vi "CRYTest and Insert CRY6181 Audio Channels.vi"(11 "Hardware in":T1={"Name"="", "Analog I/O"=0, "Digital I/O"=0, "Channels"=2, "Dig Dev ID"=1, "N ports"=3, "Interface"=0, "Dig I/O Ports"=[{"port #"=1, "width"=8, "direction"=0}, {"port #"=2, "width"=8, "direction"=0}, {"port #"=3, "width"=8, "direction"=0}], "Interf settings"=[], "N interfs"=3, "udev SNs"=[], "udev enable"=FALSE, "Channel Array"=[], "Cal sequence"="", "SelectedIn"=0, "SelectedOut"=0, "SelectedTab"=0, "State"=FALSE, "Help"="", "Advanced"=FALSE, "In Audio Driver"=0, "Out Audio Driver"=0} {"Channel Array"."Coupling" items=["Default"=-1, "RSE"=10083, "NRSE"=10078, "Differential"=10106, "Pseudodifferential"=12529]; "Channel Array"."term config" items=["Default"=-1, "RSE"=10083, "NRSE"=10078, "Differential"=10106, "Pseudodifferential"=12529]; "Channel Array"."Anti-aliasing Factor (%fs)" format="%.2f"}) -> (0 "Inserted channels":bool, 3 "Hardware out":T1={"Name"="", "Analog I/O"=0, "Digital I/O"=0, "Channels"=2, "Dig Dev ID"=1, "N ports"=3, "Interface"=0, "Dig I/O Ports"=[{"port #"=1, "width"=8, "direction"=0}, {"port #"=2, "width"=8, "direction"=0}, {"port #"=3, "width"=8, "direction"=0}], "Interf settings"=[], "N interfs"=3, "udev SNs"=[], "udev enable"=FALSE, "Channel Array"=[], "Cal sequence"="", "SelectedIn"=0, "SelectedOut"=0, "SelectedTab"=0, "State"=FALSE, "Help"="", "Advanced"=FALSE, "In Audio Driver"=0, "Out Audio Driver"=0} {"Channel Array"."Coupling" items=["Default"=-1, "RSE"=10083, "NRSE"=10078, "Differential"=10106, "Pseudodifferential"=12529]; "Channel Array"."term config" items=["Default"=-1, "RSE"=10083, "NRSE"=10078, "Differential"=10106, "Pseudodifferential"=12529]; "Channel Array"."Anti-aliasing Factor (%fs)" format="%.2f"})   [LabVIEW 2013]
uses:
  Typedef Control/CRYHardware.ctl
  Typedef Control/CRYHardware Channel Info.ctl
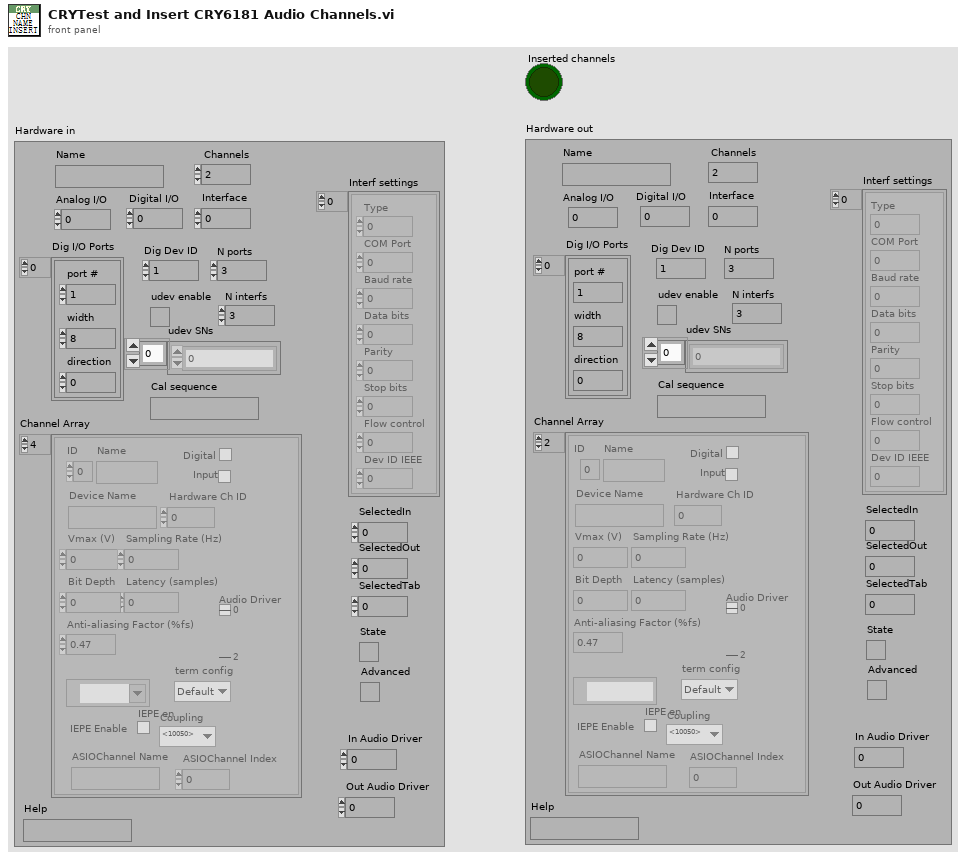
[diagram p1: front panel]
types:
  T1 = typedef "CRYHardware.ctl" = cluster{"Name":string, "Analog I/O":u16, "Digital I/O":u16, "Channels":u8, "Dig Dev ID":u8, "N ports":u8, "Interface":u32, "Dig I/O Ports":cluster{"port #":i16, "width":i16, "direction":i32}[], "Interf settings":cluster{"Type":u16, "COM Port":u8, "Baud rate":u32, "Data bits":u32, "Parity":u16, "Stop bits":u16, "Flow control":u16, "Dev ID IEEE":u8}[], "N interfs":i32, "udev SNs":i16[], "udev enable":bool, "Channel Array":T2[], "Cal sequence":string, "SelectedIn":u16, "SelectedOut":u16, "SelectedTab":u16, "State":bool, "Help":string, "Advanced":bool, "In Audio Driver":u16, "Out Audio Driver":u16}
  T2 = typedef "CRYHardware Channel Info.ctl" = cluster{"ID":i32, "Name":string, "Digital":bool, "Input":bool, "Device Name":string, "Hardware Ch ID":u8, "Vmax (V)":dbl, "Latency (samples)":dbl, "Sampling Rate (Hz)":u32, "Bit Depth":u32, "Anti-aliasing Factor (%fs)":sgl, "DAQmx Channel":tag, "term config":i32, "Coupling":i32, "IEPE en":bool, "ASIOChannel Name":string, "Audio Driver":u16, "ASIOChannel Index":u8}
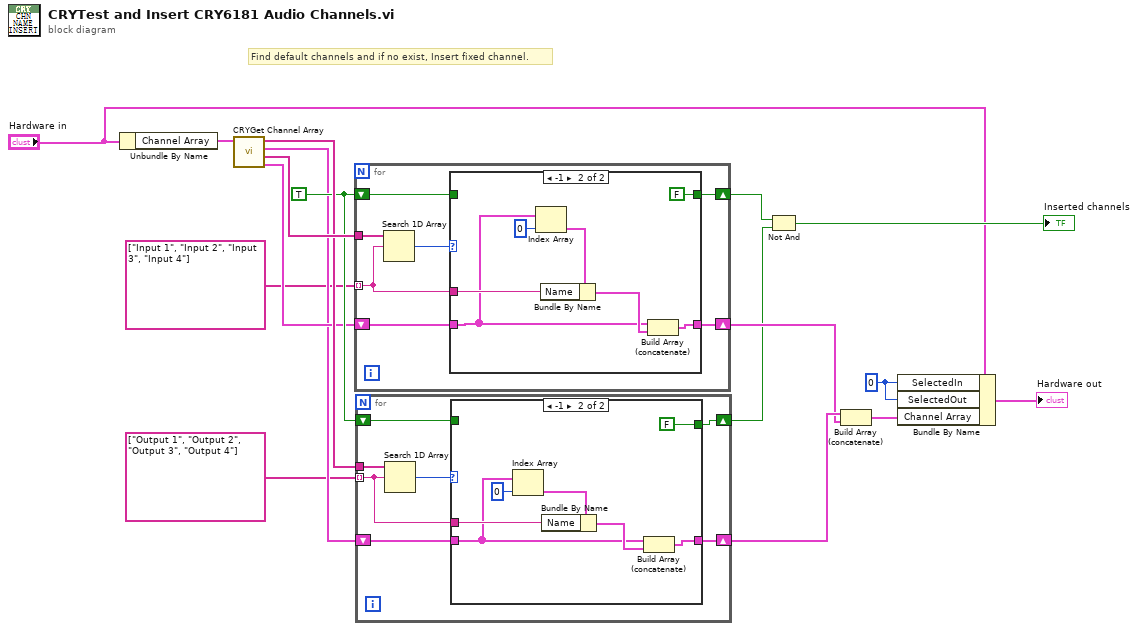
[diagram p0: block diagram]
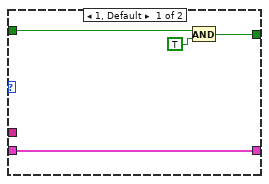
[diagram p2: hidden frame]
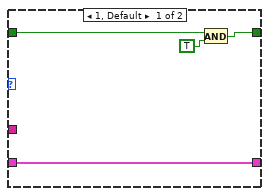
[diagram p3: hidden frame]
diagram:
  w8 = TRUE
  w11 = u16 0 ("SelectedIn")
  # "Find default channels and if no exist, Insert fixed channel."
  n1 = Unbundle By Name("Hardware in") -> ("Channel Array"=w17:T2[])
  n2 = call "CRYGet Channel Array.vi"("Channel Array"=w17) -> ("I Channel Info Out"=w7:T2[], "I_Channel Name Out"=w16:string[], "O Channel Info Out"=w6:T2[], "O_Channel Name Out"=w15:string[])  [unwired: 7 in]
  n3 = for {
    tunnel: string[] ["Input 1", "Input 2", "Input 3", "Input 4"] -> [w22] mode=indexing
    tunnel: w16 -> [w23]
    shift-right: [w24] -> w13
    shift-left: w7 -> [w20]
    shift-right: [w18] -> w9
    shift-left: w8 -> [w19]
    n4 = Search 1D Array(1D array=w23, element=w22) -> (index of element=w21:i32)  [unwired: 1 in]
    n5 = case shown="-1" w21 {
      tunnel: [w25 w32] -> w24
      tunnel: w22 -> [_ w35]
      tunnel: w20 -> [w25 w29]
      tunnel: w19 -> [w28 _]
      tunnel: [w26 FALSE ("x .and. y?")] -> w18
      frame 1, Default {
        n6 = And(x=w28, y=TRUE) -> (x .and. y?=w26:bool)
      }
      frame -1 {
        n7 = Index Array(array=w29, index=0) -> (element=w34:T2)
        n8 = Bundle By Name(cluster=w34, "Name"=w35) -> (w33:T2)
        n9 = Build Array (concatenate)(w29, w33) -> (w32:T2[])
      }
    }
  }
  n10 = for {
    tunnel: string[] ["Output 1", "Output 2", "Output 3", "Output 4"] -> [w40] mode=indexing
    tunnel: w15 -> [w41]
    shift-right: [w42] -> w14
    shift-left: w6 -> [w38]
    shift-right: [w36] -> w10
    shift-left: w8 -> [w37]
    n11 = Search 1D Array(1D array=w41, element=w40) -> (index of element=w39:i32)  [unwired: 1 in]
    n12 = case shown="-1" w39 {
      tunnel: [w43 w50] -> w42
      tunnel: w40 -> [_ w53]
      tunnel: w38 -> [w43 w47]
      tunnel: w37 -> [w45 _]
      tunnel: [w44 FALSE] -> w36
      frame 1, Default {
        n13 = And(x=w45, y=TRUE) -> (x .and. y?=w44:bool)
      }
      frame -1 {
        n14 = Index Array(array=w47, index=0) -> (element=w52:T2)
        n15 = Bundle By Name(cluster=w52, "Name"=w53) -> (w51:T2)
        n16 = Build Array (concatenate)(w47, w51) -> (w50:T2[])
      }
    }
  }
  n17 = Not And(1:w10, 2:w9) -> (0:→"Inserted channels":bool)
  n18 = Build Array (concatenate)(w14, w13) -> (w12:T2[])
  n19 = Bundle By Name(cluster="Hardware in", "SelectedIn"=w11, "SelectedOut"=w11, "Channel Array"=w12) -> (→"Hardware out":T1)
